vi "SMBus Get Alert.vi"(8 "error in (no error)":errorcluster, 9 "SMBUSIndex":i32, 10 "DevIndex":i32, 11 "DevType":i32) -> (0 "error out":errorcluster, 2 "function return":i32, 3 "pAlertFlag":string)   [LabVIEW 2012, in "ControlSMBus.lvlib"]
doc: "int WINAPI SMBus_GetAlert(int DevType,int DevIndex,int SMBUSIndex,unsigned char *pAlertFlag);"
uses:
  ControlSMBus.lvlib
  Ginkgo_Driver.dll
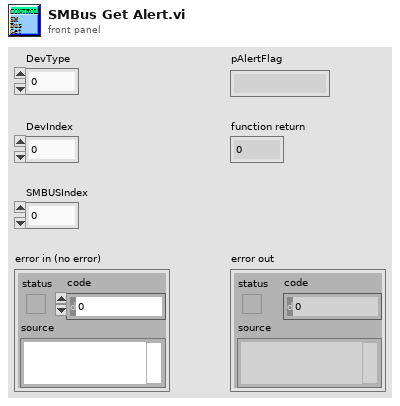
[diagram p1: front panel]
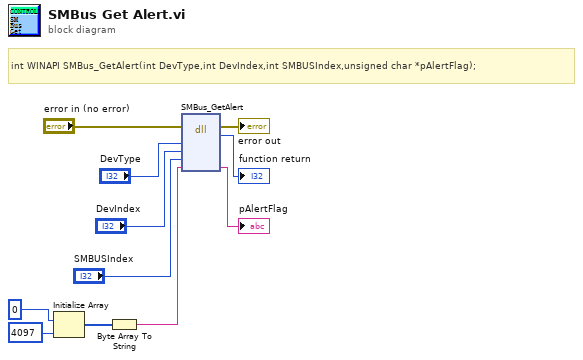
[diagram p0: block diagram]
diagram:
  # "int WINAPI SMBus_GetAlert(int DevType,int DevIndex,int SMBUSIndex,unsigned char *pAlertFlag);"
  n1 = Initialize Array(u8 0 ("element"), 4097 ("dimension size")) -> (w7:u8[])
  n2 = Byte Array To String(unsigned byte array=w7) -> (string=w6:string)
  n3 = dll-call lib="E:/Project/vt_ginkgo/truck/Ginkgo Driver/vs2010/Ginkgo_USB-I2C_API_v2.0.3.0/lib/labview_32bit/ControlSMBus/Ginkgo_Driver.*" fn="SMBus_GetAlert"(error in="error in (no error)", "DevType"="DevType", "DevIndex"="DevIndex", "SMBUSIndex"="SMBUSIndex", "pAlertFlag"=w6) -> (error out=→"error out":errorcluster, →"function return":i32, "pAlertFlag"=→"pAlertFlag":string)  [unwired: 5 in, 1 out]
